vi "Cryostation.Get Sample Temperature.vi"(8 "error in (no error)":errorcluster, 11 "TCP Network Connection in":refnum<k5>) -> (0 "error out":errorcluster, 2 "Sample Temperature (K)":dbl, 3 "TCP Network Connection out":refnum<k5>)   [LabVIEW 2019, in "instrument.Cryostation.lvclass"]
uses:
  instrument.Cryostation.lvclass
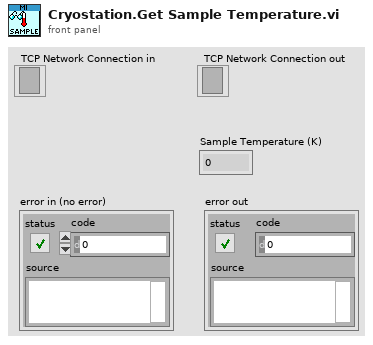
[diagram p1: front panel]
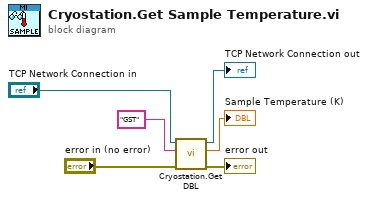
[diagram p0: block diagram]
diagram:
  n1 = call "Cryostation.Get DBL.vi"("error in (no error)"="error in (no error)", "Command"="GST", "connection ID in"="TCP Network Connection in") -> ("error out"=→"error out":errorcluster, "Response"=→"Sample Temperature (K)":dbl, "connection ID out"=→"TCP Network Connection out":refnum<k5>)  [unwired: 6 in]
